vi "Old Drive Measure Encoder Speed.vi"   [LabVIEW 2009]
uses:
  Drive Control Global.vi
  Motor Control Global.vi
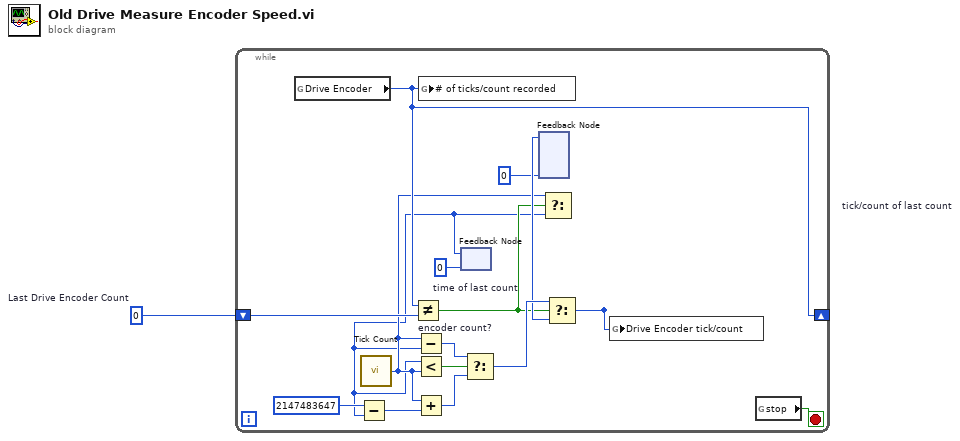
[diagram p0: block diagram]
diagram:
  w1 = 0  # Last Drive Encoder Count
  n1 = while {
    shift-right: [w15] -> _
    shift-left: w1 -> [w16]
    stop <- w17 stop-if-true
    n2 = global read "Motor Control Global.vi" "Drive Encoder"() -> (w15:i32)
    n3 = call "Tick Count"() -> ("Tick Count(Ticks)"=w5:u32)
    n4 = Not Equal? "encoder count?"(x=w15, y=w16) -> (x != y?=w6:bool)
    n5 = global write "Drive Control Global.vi" "# of ticks/count recorded"(w15) -> ()
    n6 = feedback #1 "time of last count"(u32 0 ("Tick Count(Ticks)")) -> (w2:u32)
    n7 = Subtract(x=u32 2147483647, y=w2) -> (x-y=w13:u32)
    n8 = Subtract(x=w5, y=w2) -> (x-y=w12:u32)
    n9 = Less?(x=w2, y=w5) -> (x < y?=w7:bool)
    n10 = Add(x=w5, y=w13) -> (x+y=w11:u32)
    n11 = Select(t=w12, s=w7, f=w11) -> (s? t:f=w10:u32)
    n12 = feedback #2 "tick/count of last count"(u32 0) -> (w9:u32)
    n13 = Select(t=w5, s=w6, f=w2) -> (s? t:f=w3:u32)
    n14 = Select(t=w10, s=w6, f=w9) -> (s? t:f=w18:u32)
    n15 = global write "Drive Control Global.vi" "Drive Encoder tick/count"(w18) -> ()
    n16 = global read "Motor Control Global.vi" "stop"() -> (w17:bool)
  }
